vi "Reshape ICCD Parameter Table.vi"(4 "Remove empty rows (F)?":bool, 6 "Remove empty columns (F)?":bool, 8 "Error In":errorcluster, 9 "Save ASCII File? (F)":bool, 10 "Repeat multicell values (F)?":bool, 11 "XLSX File":path) -> (0 "Error Out":errorcluster, 1 "Parameter Values":cluster{"Parameter":string, "Values":string[]}[](array[cluster]), 2 "ICCD Parameter Array":string[][](array[string]), 3 "Header":string[](array[string]))   [LabVIEW 2021, in "AlliGator Camera Noise Influence on Lifetime.lvlib"]
uses:
  AlliGator Camera Noise Influence on Lifetime.lvlib
  ICCD Parameter Value List.ctl
  0763977d-2977-455b-967a-d7a185485925.vi
  5e3e18dc-f85e-4238-93e2-d28850a51d9b.vi
  <userlib>/_OpenG.lib/array/array.llb/Remove Duplicates from 1D Array (String)__ogtk.vi
  <vilib>/Utility/file.llb/Write Delimited Spreadsheet (string).vi
  <vilib>/Comparison/Less/Less Functor/Less Functor.lvclass
  Files/Files.lvlib
  <userlib>/_OpenG.lib/array/array.llb/openg_array.lvlib
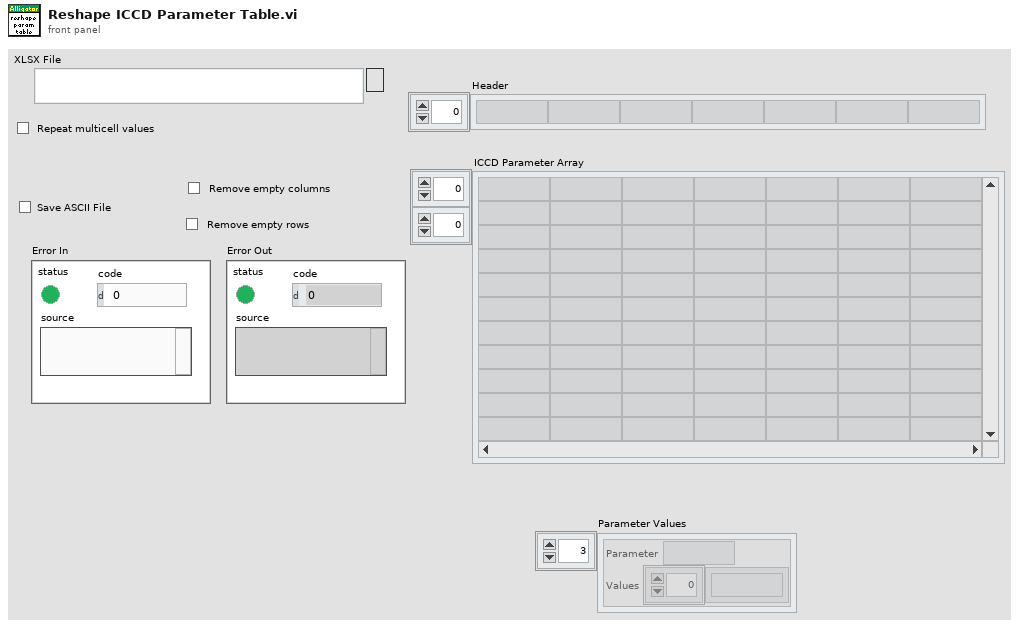
[diagram p1: front panel]
types:
  T1 = typedef "AlliGator Camera Noise Influence on Lifetime.lvlib/ICCD Parameter Value List.ctl" = cluster{"Parameter":string, "Values":string[]}
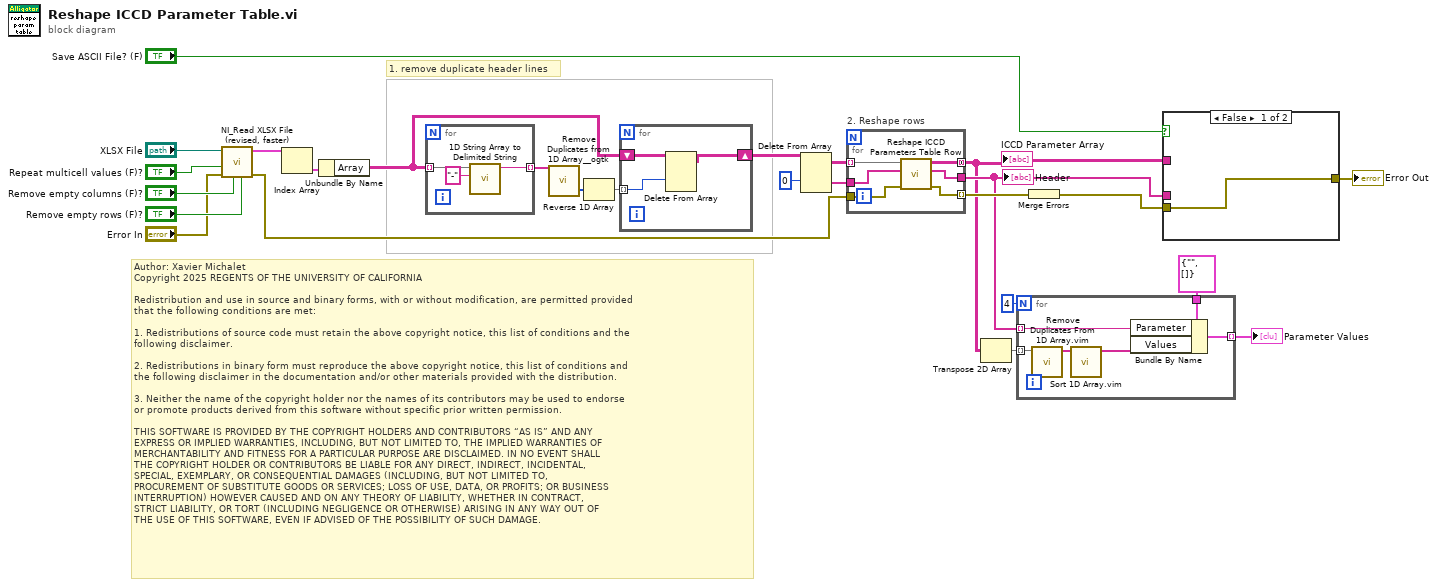
[diagram p0: block diagram]
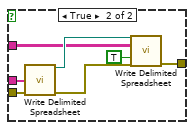
[diagram p2: hidden frame]
diagram:
  # "Author: Xavier Michalet\nCopyright 2025 REGENTS OF THE UNIVERSITY OF CALIFORNIA\n\nRedistribution and use in source and binary forms, with or without modification, are permitted provided\nthat the following conditions are met:\n\n1. Redistributions of source code must retain the above copyright notice, this list of conditions and the\nfollowing disclaimer.\n\n2. Redistributions in binary form must reproduce the above copyright notice, this list of conditions and\nthe following disclaimer in the documentation and/or other materials provided with the distribution.\n\n3. Neither the name of the copyright holder nor the names of its contributors may be used to endorse \nor promote products derived from this software without specific prior written permission.\n\nTHIS SOFTWARE IS PROVIDED BY THE COPYRIGHT HOLDERS AND CONTRIBUTORS “AS IS” AND ANY \nEXPRESS OR IMPLIED WARRANTIES, INCLUDING, BUT NOT LIMITED TO, THE IMPLIED WARRANTIES OF\nMERCHANTABILITY AND FITNESS FOR A PARTICULAR PURPOSE ARE DISCLAIMED. IN NO EVENT SHALL\nTHE COPYRIGHT HOLDER OR CONTRIBUTORS BE LIABLE FOR ANY DIRECT, INDIRECT, INCIDENTAL, \nSPECIAL, EXEMPLARY, OR CONSEQUENTIAL DAMAGES (INCLUDING, BUT NOT LIMITED TO, \nPROCUREMENT OF SUBSTITUTE GOODS OR SERVICES; LOSS OF USE, DATA, OR PROFITS; OR BUSINESS\nINTERRUPTION) HOWEVER CAUSED AND ON ANY THEORY OF LIABILITY, WHETHER IN CONTRACT, \nSTRICT LIABILITY, OR TORT (INCLUDING NEGLIGENCE OR OTHERWISE) ARISING IN ANY WAY OUT OF\nTHE USE OF THIS SOFTWARE, EVEN IF ADVISED OF THE POSSIBILITY OF SUCH DAMAGE."
  # "1. remove duplicate header lines"
  n1 = call "NI_Read XLSX File (revised, faster).vi"("Remove empty rows"="Remove empty rows (F)?", "Remove empty columns"="Remove empty columns (F)?", "error in"="Error In", "Repeat multicell values"="Repeat multicell values (F)?", "XLSX File"="XLSX File") -> ("error out"=w13:errorcluster, "Sheet Data"=w22:cluster{"Array":string[][]}[])  [unwired: 4 in, 1 out]
  n2 = Index Array(array=w22) -> (element=w21:cluster{"Array":string[][]})  [unwired: 1 in]
  n3 = Unbundle By Name(w21) -> ("Array"=w17:string[][])
  n4 = for {
    tunnel: w17 -> [w29] mode=indexing
    tunnel: [w28] -> w20 mode=indexing
    n5 = call <vilib>:"1D String Array to Delimited String.vi"("delimiter"="-", "string array"=w29) -> ("delimited string"=w28:string)  [unwired: 9 in]
  }
  n6 = call-poly <userlib>:"Remove Duplicates from 1D Array__ogtk.vi"("Input Array"=w20) -> ("indices of removed elements"=w19:i32[])  [unwired: 1 out]
  n7 = Reverse 1D Array(array=w19) -> (reversed array=w18:i32[])
  n8 = for {
    tunnel: w18 -> [w31] mode=indexing
    shift-right: [w30] -> w15
    shift-left: w17 -> [w32]
    n9 = Delete From Array(array=w32, index (row)=w31) -> (array with subset deleted=w30:string[][])  [unwired: 2 in, 1 out]
  }
  n10 = Delete From Array(array=w15, index (row)=0) -> (deleted portion=w16:string[], array with subset deleted=w14:string[][])  [unwired: 2 in]
  n11 = for "2. Reshape rows" {
    tunnel: w16 -> [w38]
    tunnel: w14 -> [w37] mode=indexing
    tunnel: [w36] -> w4 mode=concatenating
    tunnel: w13 -> [w35]
    tunnel: [w34] -> w6
    tunnel: [w33] -> w11 mode=indexing
    n12 = call "Reshape ICCD Parameters Table Row.vi"("error in (no error)"=w35, "Header"=w38, "Array in"=w37) -> ("error out"=w33:errorcluster, "Header out"=w34:string[], "Array out"=w36:string[][])  [unwired: 6 in]
  }
  "ICCD Parameter Array" <- w4
  "Header" <- w6
  n13 = Transpose 2D Array(2D array=w4) -> (transposed array=w3:string[][])
  n14 = for {
    N: 4 -> [_]
    tunnel: w6 -> [w44] mode=indexing
    tunnel: T1 {"Parameter"="", "Values"=[]} ("Parameter Values") -> [w43]
    tunnel: w3 -> [w42] mode=indexing
    tunnel: [w39] -> w2 mode=indexing
    n15 = call "Remove Duplicates From 1D Array.vim"("array"=w42) -> ("array with duplicates removed"=w41:string[])  [unwired: 10 in]
    n16 = call "Sort 1D Array.vim"("unsorted array"=w41) -> ("sorted array"=w40:string[])  [unwired: 10 in]
    n17 = Bundle By Name(cluster=w43, "Parameter"=w44, "Values"=w40) -> (w39:T1)
  }
  "Parameter Values" <- w2
  n18 = Merge Errors(w11) -> (w10:errorcluster)
  n19 = case shown="False" "Save ASCII File? (F)" {
    tunnel: w10 -> [w45 w51]
    tunnel: [w45 w48] -> w8
    tunnel: w6 -> [_ w47]
    tunnel: w4 -> [_ w46]
    frame False {
    }
    frame True {
      n20 = call-poly <vilib>:"Write Delimited Spreadsheet.vi"("1D data"=w47, "error in (no error)"=w51) -> ("new file path (Not A Path if cancelled)"=w49:path, "error out"=w50:errorcluster)  [unwired: 12 in]
      n21 = call-poly <vilib>:"Write Delimited Spreadsheet.vi"("file path (dialog if empty)"=w49, "2D data"=w46, "append to file? (new file:F)"=TRUE, "error in (no error)"=w50) -> ("error out"=w48:errorcluster)  [unwired: 10 in, 1 out]
    }
  }
  "Error Out" <- w8
